vi "Path Keeper_Write Path to INI.vi"(8 "Error In":errorcluster, 9 "File / Directory Name In":string, 10 "Path In":path, 11 "Ini Ref In":T1) -> (0 "Error Out":errorcluster, 2 "Path Out":path, 3 "Ini Ref Out":T1)   [LabVIEW 2015]
uses:
  <vilib>/Utility/config.llb/Config Data RefNum.ctl
  <vilib>/Utility/config.llb/Write Key (Path).vi
  <vilib>/Utility/config.llb/NI_LVConfig.lvlib
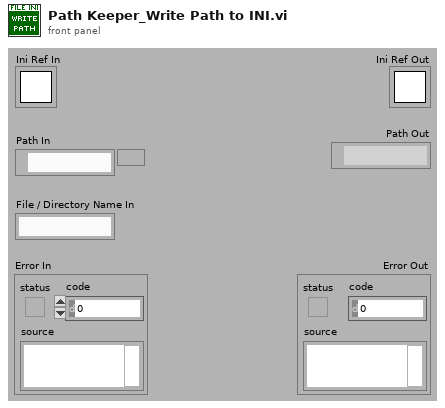
[diagram p1: front panel]
types:
  T1 = typedef "NI_LVConfig.lvlib/Config Data RefNum.ctl" = refnum<k1>
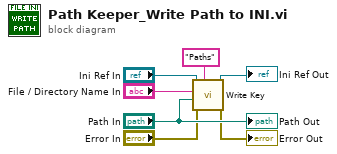
[diagram p0: block diagram]
diagram:
  n1 = call-poly <vilib>:"Write Key.vi"("section"="Paths", "error in (no error)"="Error In", "value"="Path In", "key"="File / Directory Name In", "refnum"="Ini Ref In") -> ("error out"=→"Error Out":errorcluster, "refnum out"=→"Ini Ref Out":T1)  [unwired: 4 in, 1 out]
  "Path Out" <- "Path In"
